vi "get file size.vi"(0 "file path":path) -> (14 "size (in bytes)":i64)   [LabVIEW 2016, in "update.lvlib" / "http client.lvclass"]
uses:
  http client.lvclass
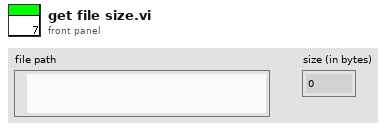
[diagram p1: front panel]
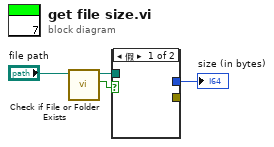
[diagram p0: block diagram]
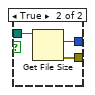
[diagram p2: hidden frame]
diagram:
  n1 = call <vilib>:"Check if File or Folder Exists.vi"("path"="file path") -> ("file or folder exists?"=w3:bool, "dup path"=w4:path)  [unwired: 8 in, 1 out]
  n2 = case shown="假" w3 {
    tunnel: [_ w7] -> w1
    tunnel: [_ w6] -> _
    tunnel: w4 -> [_ w5]
    frame False {
    }
    frame True {
      n3 = Get File Size(file=w5) -> (size (in bytes)=w7:i64, 0:w6:errorcluster)  [unwired: 1 in, 1 out]
    }
  }
  "size (in bytes)" <- w1
